vi "全局文件路径常量.vi"(8 "error in (no error)":errorcluster caption="错误输入（无错误）") -> (0 "error out":errorcluster, 2 "Email服务器配置":path, 3 "用户数据库根目录":path)   [LabVIEW 2013, in "个人剂量仪-云服务器.lvclass"]
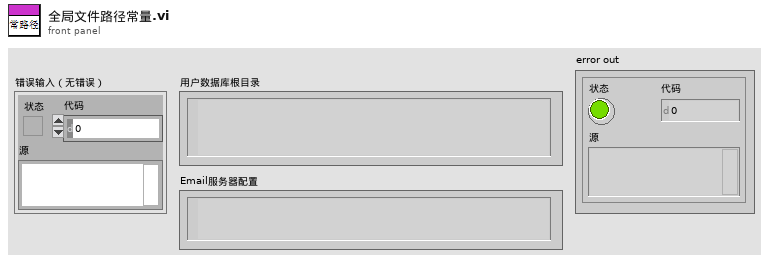
[diagram p1: front panel]
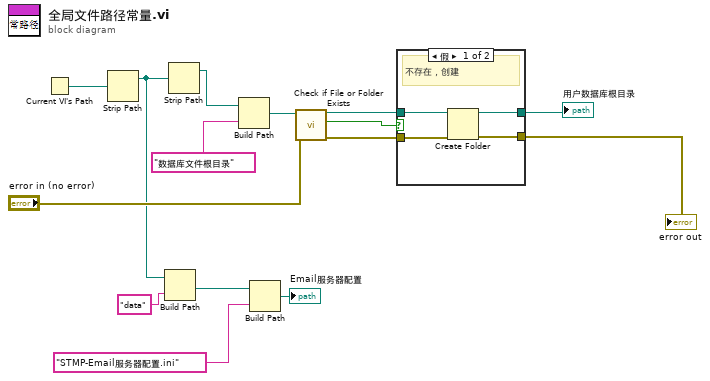
[diagram p0: block diagram]
diagram:
  n1 = Current VI's Path() -> (path=w15:path)
  n2 = Strip Path(path=w15) -> (stripped path=w5:path)  [unwired: 1 out]
  n3 = Build Path(base path=w5, name or relative path="data" ("名称或相对路径")) -> (appended path=w3:path)
  n4 = Strip Path(path=w5) -> (stripped path=w14:path)  [unwired: 1 out]
  n5 = Build Path(base path=w14, name or relative path="数据库文件根目录" ("名称或相对路径")) -> (appended path=w12:path)
  n6 = Build Path(base path=w3, name or relative path="STMP-Email服务器配置.ini" ("名称或相对路径")) -> (appended path=→"Email服务器配置":path)
  n7 = call <vilib>:"Check if File or Folder Exists.vi"("error in (no error)"="error in (no error)", "path"=w12) -> ("error out"=w7:errorcluster, "file or folder exists?"=w11:bool, "dup path"=w10:path)  [unwired: 7 in]
  n8 = case shown="假" w11 {
    tunnel: w10 -> [w19 w21]
    tunnel: [w18 w21] -> w9
    tunnel: w7 -> [w17 w20]
    tunnel: [w16 w20] -> w6
    frame False {
      # "不存在，创建"
      n9 = Create Folder(path (use dialog)=w19, error in=w17) -> (created path=w18:path, error out=w16:errorcluster)  [unwired: 1 in, 1 out]
    }
    frame True {
      # "已存在"
    }
  }
  "用户数据库根目录" <- w9
  "error out" <- w6
